vi "GVSView Pic Out Log.vi"(6 "vi reference":refnum<vi>, 11 "sData":string) -> ()   [LabVIEW 2013]
uses:
  SubVI/GVSMain Sub Window Global.vi
  GVSView Global.vi
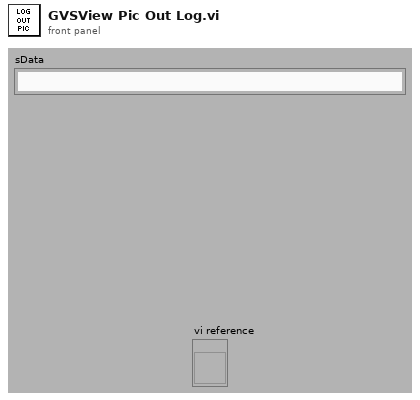
[diagram p1: front panel]
types:
  T1 = enum16{"open", "open or create", "create or replace", "create", "open (read only)"}
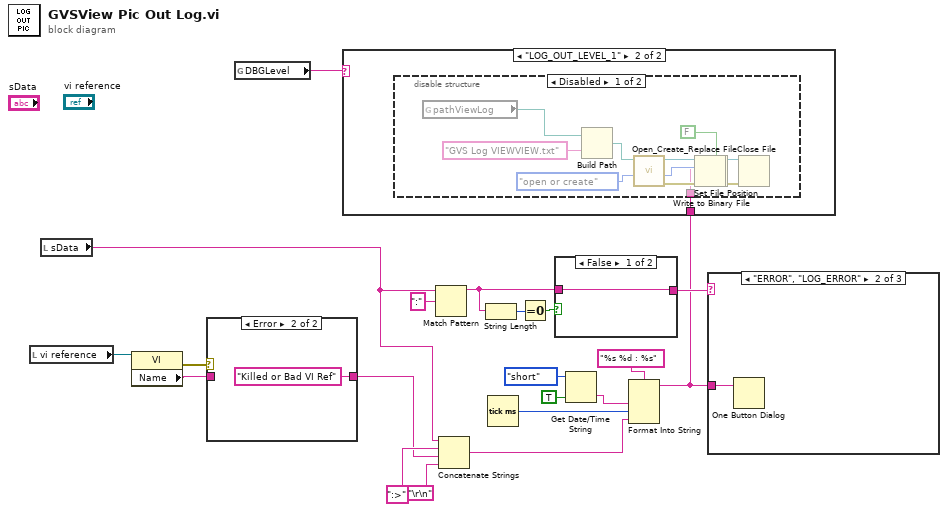
[diagram p0: block diagram]
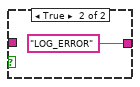
[diagram p5: hidden frame]
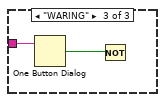
[diagram p7: hidden frame]
diagram:
  n1 = local read "vi reference"() -> (w20:refnum<vi>)
  n2 = local read "sData"() -> (w16:string)
  n3 = property class="VI"(reference=w20) -> (error out=w10:errorcluster, "Name"=w9:string)  [unwired: 1 in, 1 out]
  n4 = case shown="Error" w10 {
    tunnel: w9 -> [w21 _]
    tunnel: [w21 "Killed or Bad VI Ref" ("Name")] -> w15
    frame No Error {
    }
    frame Error {
    }
  }
  n5 = global read "GVSMain Sub Window Global.vi" "DBGLevel"() -> (w1:string)
  n6 = Match Pattern(string=w16, regular expression=":") -> (before substring=w12:string)  [unwired: 1 in, 3 out]
  n7 = Concatenate Strings(w16, ":>" ("string"), w15, "\r\n") -> (w3:string)
  n8 = String Length(string=w12) -> (length=w14:i32)
  n9 = Tick Count (ms)() -> (millisecond timer value=w4:u32)
  n10 = Equal To 0?(x=w14) -> (x = 0?=w13:bool)
  n11 = case shown="False" w13 {
    tunnel: [w23 "LOG_ERROR" ("sData")] -> w11
    tunnel: w12 -> [w23 _]
    frame False {
    }
    frame True {
    }
  }
  n12 = Get Date/Time String(date format (0)=enum16{"short", "long", "abbreviated"}."short", want seconds? (F)=TRUE) -> (time string=w5:string)  [unwired: 1 in, 1 out]
  n13 = Format Into String(format string="%s %d : %s", w5, w4, w3) -> (resulting string=w2:string)  [unwired: 2 in, 1 out]
  n14 = case shown="\"LOG_OUT_LEVEL_1\"" w1 {
    tunnel: w2 -> [_ w25]
    frame Default {
    }
    frame "LOG_OUT_LEVEL_1" {
      n15 = disable-structure shown="Disabled" {
        disable-tunnel: w25 -> [w26 _]
        frame Disabled {
          n16 = global read "GVSView Global.vi" "pathViewLog"() -> (w27:path)
          n17 = Build Path(base path=w27, name or relative path="GVS Log VIEWVIEW.txt" ("name")) -> (appended path=w28:path)
          n18 = call <vilib>:"Open_Create_Replace File.vi"("function (open:0)"=T1."open or create", "file path"=w28) -> ("error out"=w36:errorcluster, "file size (bytes)"=w34:i32, "refnum"=w35:refnum<file>)  [unwired: 6 in, 1 out]
          n19 = Set File Position(offset (in bytes) (0)=w34, refnum=w35, error in=w36) -> (refnum out=w31:refnum<file>, error out=w30:errorcluster)  [unwired: 1 in]
          n20 = Write to Binary File(file (use dialog)=w31, data=w26, error in=w30, 5:FALSE ("prepend array or string size? (T)")) -> (refnum out=w32:refnum<file>, error out=w33:errorcluster)  [unwired: 2 in, 1 out]
          n21 = Close File(refnum=w32, error in=w33) -> ()  [unwired: 2 out]
        }
        frame Enabled {
        }
      }
    }
  }
  n22 = case shown="\"ERROR\", \"LOG_ERROR\"" w11 {
    tunnel: w2 -> [_ w39 w40]
    frame Default {
    }
    frame "ERROR", "LOG_ERROR" {
      n23 = One Button Dialog(message=w39) -> ()  [unwired: 1 in, 1 out]
    }
    frame "WARING" {
      n24 = One Button Dialog(message=w40) -> (true=w41:bool)  [unwired: 1 in]
      n25 = Not(x=w41) -> ()  [unwired: 1 out]
    }
  }
